vi "LJUD_StringToConstant.vi"(8 "error in":errorcluster, 11 "String":string) -> (0 "error out":errorcluster, 3 "Constant Number":i32)   [LabVIEW 2020]
doc: "Converts the given string to the appropriate constant\nnumber. Used internally by the S functions.\n\nDocumented in Section 4.2 of the device's datasheet."
uses:
  labjackud.dll
panel:
  # "Converts the given string to the appropriate constant\nnumber. Used internally by the S functions.\n\nDocumented in Section 4.2 of the device's datasheet."
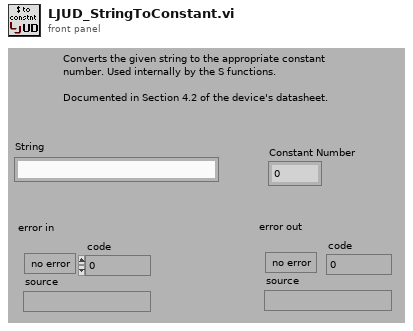
[diagram p1: front panel]
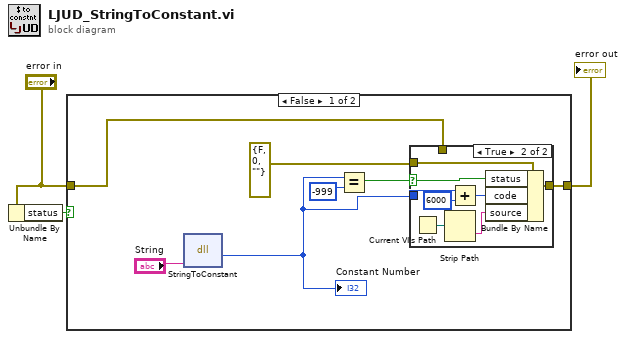
[diagram p0: block diagram]
diagram:
  n1 = Unbundle By Name("error in") -> ("status"=w1:bool)
  n2 = case shown="False" w1 {
    tunnel: [w8 w20] -> w3
    tunnel: "error in" -> [w4 w20]
    frame False {
      n3 = dll-call lib="labjackud.dll" fn="StringToConstant"("String"="String") -> (w5:i32)  [unwired: 4 in, 2 out]
      "Constant Number" <- w5
      n4 = Equal?(x=w5, y=-999) -> (x = y?=w6:bool)
      n5 = case shown="True" w6 {
        selector: w6 -> [_ w18]
        tunnel: [w11 w19] -> w8
        tunnel: errorcluster {"status"=FALSE, "code"=0, "source"=""} ("error IO") -> [_ w17]
        tunnel: w5 -> [_ w13]
        tunnel: w4 -> [w11 _]
        frame False {
        }
        frame True {
          n6 = Current VI's Path() -> (path=w15:path)
          n7 = Strip Path(path=w15) -> (name=w16:string)  [unwired: 1 out]
          n8 = Add(x=w13, y=6000) -> (x+y=w14:i32)
          n9 = Bundle By Name(cluster=w17, "status"=w18, "code"=w14, "source"=w16) -> (w19:errorcluster)
        }
      }
    }
    frame True {
    }
  }
  "error out" <- w3
